vi "ComputeZ.vi"(2 "angular_steps":i32=64, 3 "position":cluster{"X":sgl, "Y":sgl}, 4 "tracker":u64) -> (0 "Z":sgl, 1 "tracker":u64)   [LabVIEW 2011]
uses:
  TrackerDLL.vi
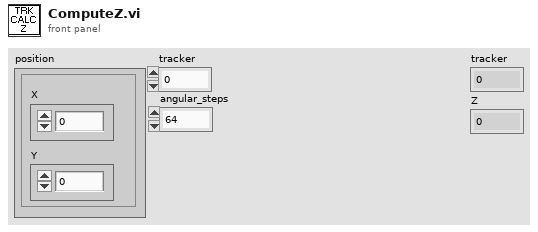
[diagram p1: front panel]
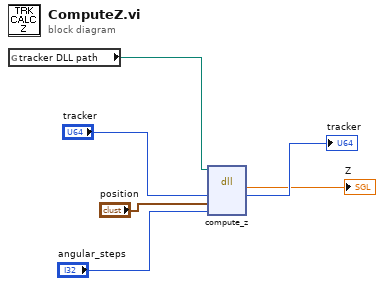
[diagram p0: block diagram]
diagram:
  n1 = global read "TrackerDLL.vi" "tracker DLL path"() -> (w3:path)
  n2 = dll-call lib="D:/jcnossen1/cudaqi-tracker/cudatrack-labview/cputrack_d.dll" fn="compute_z"(path in=w3, "tracker"="tracker", "center"="position", "angular_steps"="angular_steps") -> ("return type"=→"Z":sgl, "tracker"=→"tracker":u64)  [unwired: 4 in, 2 out]
